vi "LabviewMonitoringApplication - Copy.vi"() -> ()   [LabVIEW 2024]
uses:
  <vilib>/Utility/error.llb/Trim Whitespace One-Sided.vi
  <vilib>/Instr/_visa.llb/VISA Configure Serial Port (Instr).vi
  <vilib>/Utility/file.llb/Read Delimited Spreadsheet (DBL).vi
panel:
  out "all rows":dbl[][](array[numeric])
  out "CONTROL PANEL":enum32{"DASHBOARD", "SERIAL PORT  Settings"}(tab)
  out "Pericol pentru sanatate":u32(colorbox)
  out "Disconfort sever":u32(colorbox)
  out "Disconfort moderat":u32(colorbox)
  out "Usor discomfort":u32(colorbox)
  out "Confortabil":u32(colorbox)
  out "Snapshot data":string
  out "Waveform Chart":T1(graph)
  out "return count read":u32
  in  "STOP":bool=TRUE
  in  "milliseconds to wait":u32=1000
  out "VISA resource name out read":refnum<visa-resource-name>="COM32"
  in  "Start Measurement":bool=TRUE
  out "READ BUFFER":string
  out "Prog. Cnt":i64
  out "AdcValue":dbl
  out "R0 value (kOHm)":dbl(slide) scale=0.0..10.0 scale format="%.2f"
  out "Volatge":dbl(knob) scale=0.0..3.3
  out "Temperature °C":dbl(slide) scale=0.0..100.0 scale format="%#.2g"
  out "Humidity %":dbl(knob) scale=0.1..100.0 scale format="%#.2g"
  out "Heat Index":dbl(slide) scale=0.0..100.0
  out "iPPM_Smoke":i64(slide) scale=0.0..500.0
  out "iPPM_LPG":i64(slide) scale=0.0..100.0
  out "iPPM_CO":i64(slide) scale=0.0..400.0
  in  "Live Data / Historical Data":bool=TRUE
  in  "Temperature":bool=TRUE
  in  "Humidity":bool=TRUE
  in  "PMM_CO":bool=TRUE
  in  "HeatIndex":bool=TRUE
  in  "PMM_LPG":bool=TRUE
  in  "PMM_Smoke":bool=TRUE
  in  "Save file":bool
  in  "Refresh snapshot data":bool
  in  "file path (use dialog)":path
  out "ITU":dbl format="%#.2g"
  in  "file path (dialog if empty)":path
  out "error out read  from VISA":errorcluster={"status"=TRUE, "code"=-1073807339, "source"="VISA Read in LabviewMonitoringApplication.vi"}
  in  "VISA resource name":refnum<visa-resource-name>="COM32"
  in  "Enable Termination\nChar (T)":bool=TRUE
  in  "timeout (ms)":u32=10000
  in  "baud rate (115200)":u32=115200
  in  "byte count":u32=100
  in  "parity (0:none)":enum16{"None", "Odd", "Even", "Mark", "Space"}(ring)
  in  "data bits (8)":u16=8 min=5 max=8 step=1
  in  "termination char\n(0xA = '\\n' = LF)":u8=10 format="%.0x"
  in  "flow control (0:none)":u16(ring) items=["None", "XON/XOFF", "RTS/CTS", "XON/XOFF & RTS/CTS", "DTR/DSR", "XON/XOFF & DTR/DSR"]
  in  "stop bits (10: 1 bit)":u16(ring)=10 items=["1.0"=10, "1.5"=15, "2.0"=20]
  out "error writing file":errorcluster
  out "Snapshot line":string
  # "Select signals (for live data)"
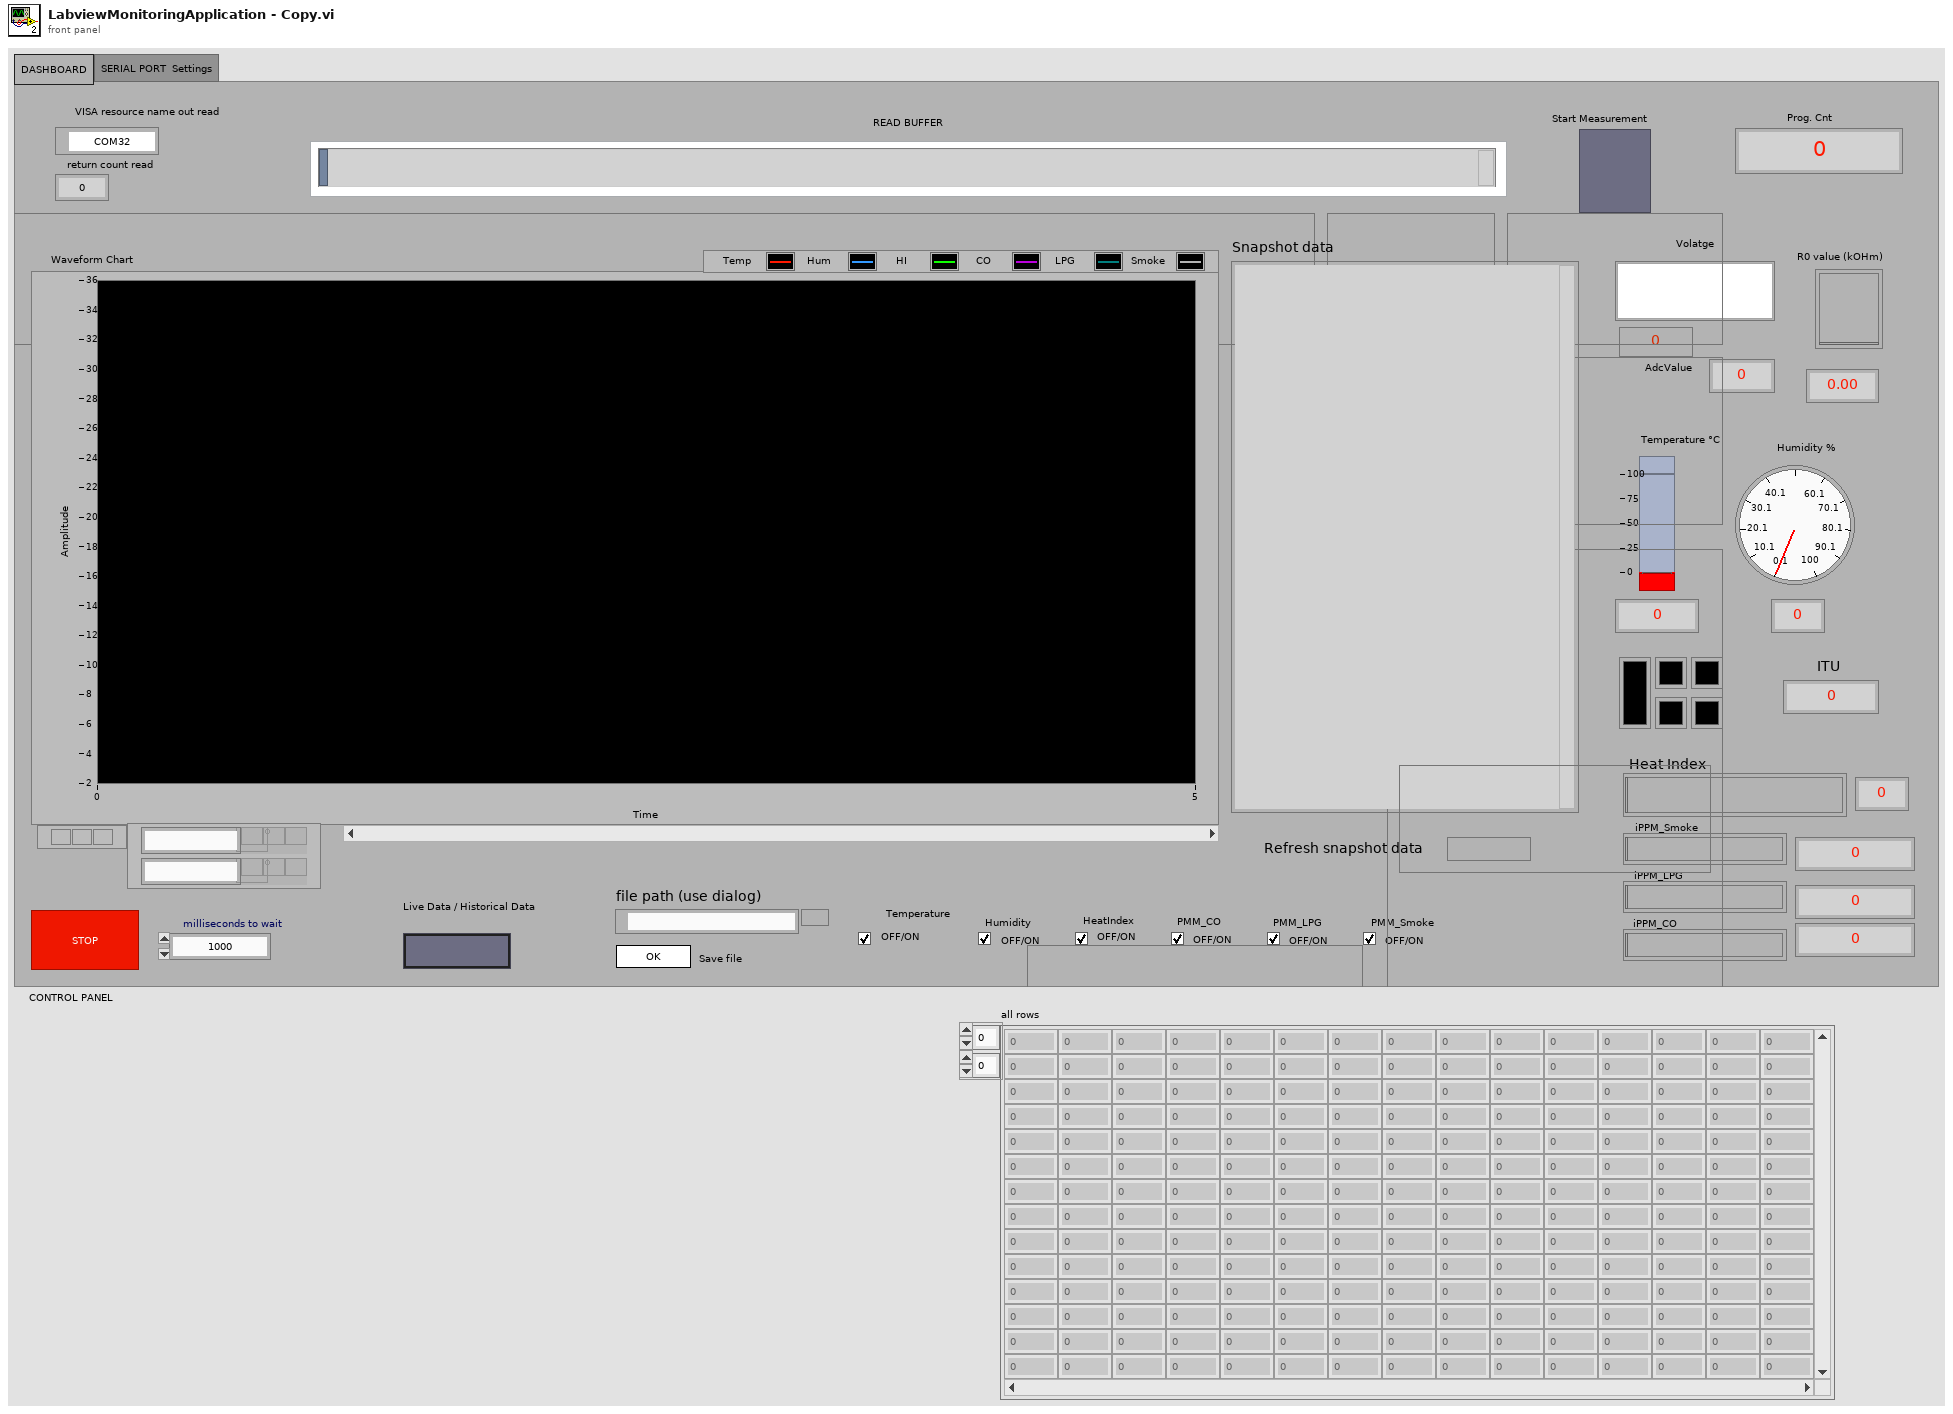
[diagram p1: front panel]
types:
  T1 = cluster{"Temperature °C ":dbl, "Humidity %":dbl, "Heat Index":dbl, "iPPM_CO":dbl, "iPPM_LPG":dbl, "iPPM_Smoke":dbl}
  T2 = enum16{"open", "replace", "create", "open or create", "replace or create", "replace or create with confirmation"}
  T3 = cluster{"Numeric":dbl, "Numeric":dbl, "Numeric":dbl, "Numeric":dbl, "Numeric":dbl, "Numeric":dbl}
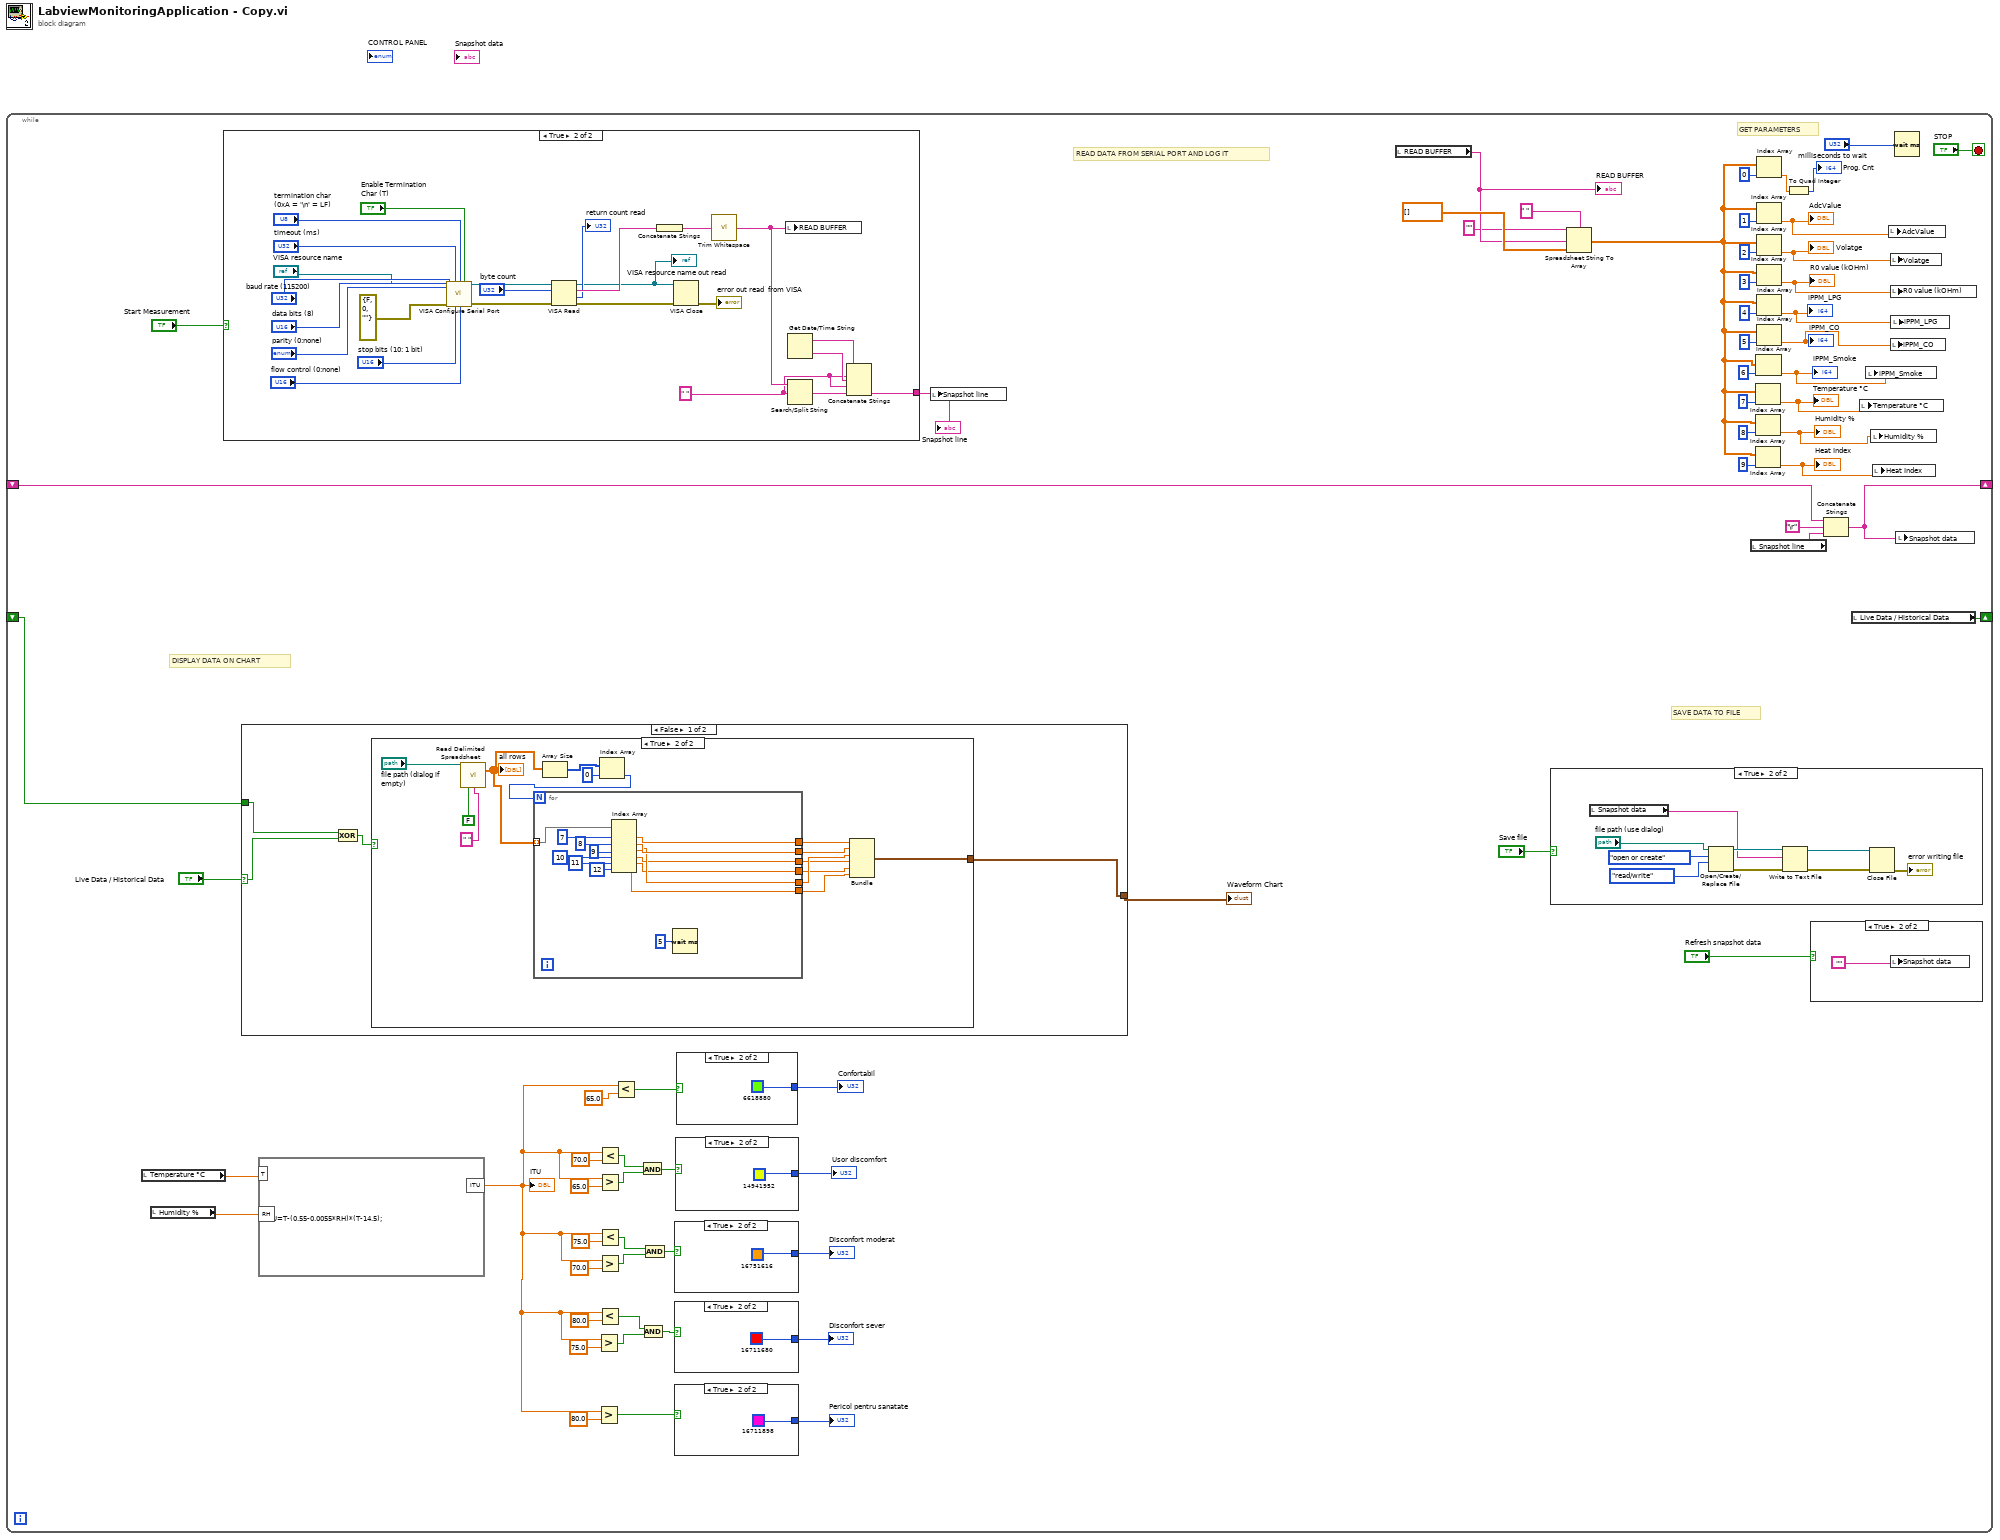
[diagram p0: block diagram]
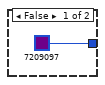
[diagram p2: hidden frame]
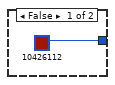
[diagram p3: hidden frame]
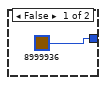
[diagram p4: hidden frame]
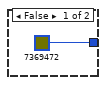
[diagram p5: hidden frame]
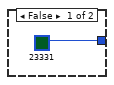
[diagram p6: hidden frame]
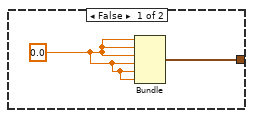
[diagram p9: hidden frame]
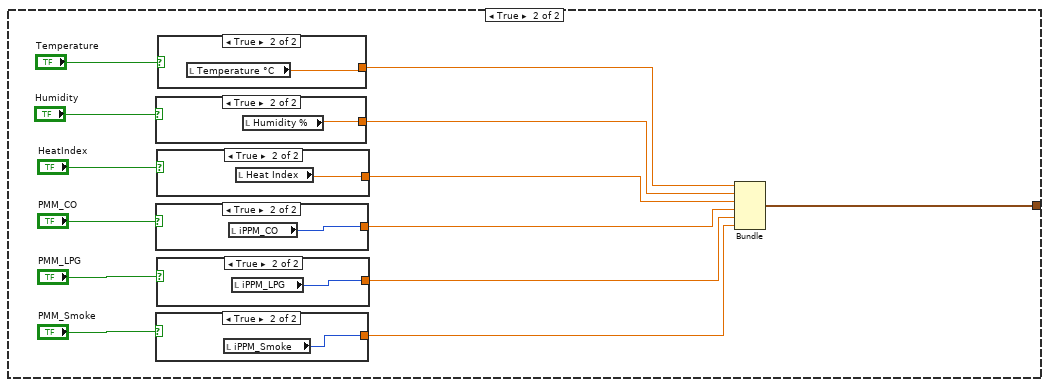
[diagram p10: hidden frame]
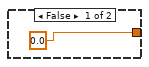
[diagram p11: hidden frame]
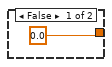
[diagram p12: hidden frame]
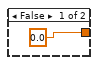
[diagram p13: hidden frame]
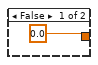
[diagram p14: hidden frame]
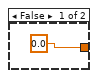
[diagram p15: hidden frame]
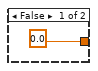
[diagram p16: hidden frame]
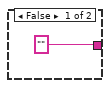
[diagram p17: hidden frame]
diagram:
  n1 = while {
    shift-right: [w33] -> _
    shift-left: _ -> [w34]
    shift-right: [w29] -> _
    shift-left: _ -> [w28]
    stop <- "STOP" stop-if-true
    # "SAVE DATA TO FILE"
    # "DISPLAY DATA ON CHART"
    # "READ DATA FROM SERIAL PORT AND LOG IT"
    # "GET PARAMETERS"
    n2 = local read "Temperature °C"() -> (w26:dbl)
    n3 = local read "Humidity %"() -> (w27:dbl)
    n4 = case shown="True" "Start Measurement" {
      tunnel: ["" w151] -> w31
      frame False {
      }
      frame True {
        w149 = " "
        n5 = call-poly "VISA Configure Serial Port"("VISA resource name"="VISA resource name", "timeout (10sec)"="timeout (ms)", "termination char\n(0xA = '\\n' = LF)"="termination char\n(0xA = '\\n' = LF)", "Enable Termination\nChar (T)"="Enable Termination\nChar (T)", "baud rate (9600)"="baud rate (115200)", "data bits (8)"="data bits (8)", "parity (0:none)"="parity (0:none)", "error in (no error)"=errorcluster {"status"=FALSE, "code"=0, "source"=""}, "stop bits (10: 1 bit)"="stop bits (10: 1 bit)", "flow control (0:none)"="flow control (0:none)") -> ("VISA resource name out"=w165:refnum<visa-resource-name>, "error out"=w164:errorcluster)  [unwired: 4 in]
        n6 = VISA Read(VISA resource name=w165, byte count="byte count", error in (no error)=w164) -> (VISA resource name out=w154:refnum<visa-resource-name>, read buffer=w163:string, return count=→"return count read":u32, error out=w155:errorcluster)
        "VISA resource name out read" <- w154
        n7 = Concatenate Strings(w163) -> (w160:string)
        n8 = VISA Close(VISA resource name=w154, error in (no error)=w155) -> (error out=→"error out read  from VISA":errorcluster)
        n9 = call <vilib>:"Trim Whitespace.vi"("string"=w160) -> ("trimmed string"=w152:string)  [unwired: 1 in]
        n10 = local write "READ BUFFER"(w152) -> ()
        n11 = Search/Split String(string=w152, search string/char (-)=w149) -> (match + rest of string=w153:string)  [unwired: 1 in, 2 out]
        n12 = Get Date/Time String() -> (date string=w148:string, time string=w150:string)  [unwired: 3 in]
        n13 = Concatenate Strings(w148, w149, w150, w149, w153) -> (w151:string)
      }
    }
    "Snapshot line" <- w31
    n14 = case shown="False" "Live Data / Historical Data" {
      selector: "Live Data / Historical Data" -> [w90 _]
      tunnel: [w88 w122] -> w38
      tunnel: w28 -> [w91 _]
      frame False {
        n15 = Exclusive Or(1:w90, 2:w91) -> (0:w89:bool)
        n16 = case shown="True" w89 {
          tunnel: [w93 w94] -> w88
          frame False {
            w92 = 0.0
            n17 = Bundle(w92, w92, w92, w92, w92, w92) -> (w93:cluster{dbl, dbl, dbl, dbl, dbl, dbl})  [unwired: 1 in]
          }
          frame True {
            n18 = call-poly <vilib>:"Read Delimited Spreadsheet.vi"("file path (dialog if empty)"="file path (dialog if empty)", "transpose? (F)"=FALSE, "delimiter (\\t)"=" ") -> ("all rows"=w101:dbl[][])  [unwired: 7 in, 5 out]
            "all rows" <- w101
            n19 = Array Size(array=w101) -> (size(s)=w103:i32[])
            n20 = Index Array(array=w103, index=0) -> (element=w102:i32)
            n21 = for {
              N: w102 -> [_]
              tunnel: w101 -> [w121] mode=indexing
              tunnel: [w114] -> w100
              tunnel: [w113] -> w99
              tunnel: [w112] -> w98
              tunnel: [w111] -> w97
              tunnel: [w110] -> w96
              tunnel: [w109] -> w95
              n22 = Index Array(array=w121, index #1=7 ("index"), index #2=8 ("index"), index #3=9 ("index"), index #4=10 ("index"), index #5=11 ("index"), index #6=12 ("index")) -> (element #1=w114:dbl, element #2=w113:dbl, element #3=w112:dbl, element #4=w111:dbl, element #5=w110:dbl, element #6=w109:dbl)
              n23 = Wait (ms)(milliseconds to wait=u32 5) -> ()  [unwired: 1 out]
            }
            n24 = Bundle("Numeric"=w100, "Numeric"=w99, "Numeric"=w98, "Numeric"=w97, "Numeric"=w96, "Numeric"=w95) -> (w94:T3)  [unwired: 1 in]
          }
        }
      }
      frame True {
        n25 = case shown="True" "Humidity" {
          tunnel: [0.0 w144] -> w127
          frame False {
          }
          frame True {
            n26 = local read "Humidity %"() -> (w144:dbl)
          }
        }
        n27 = case shown="True" "PMM_CO" {
          tunnel: [0.0 w140] -> w125
          frame False {
          }
          frame True {
            n28 = local read "iPPM_CO"() -> (w140:i64)
          }
        }
        n29 = case shown="True" "PMM_Smoke" {
          tunnel: [0.0 w136] -> w123
          frame False {
          }
          frame True {
            n30 = local read "iPPM_Smoke"() -> (w136:i64)
          }
        }
        n31 = case shown="True" "HeatIndex" {
          tunnel: [0.0 w142] -> w126
          frame False {
          }
          frame True {
            n32 = local read "Heat Index"() -> (w142:dbl)
          }
        }
        n33 = case shown="True" "PMM_LPG" {
          tunnel: [0.0 w138] -> w124
          frame False {
          }
          frame True {
            n34 = local read "iPPM_LPG"() -> (w138:i64)
          }
        }
        n35 = case shown="True" "Temperature" {
          tunnel: [0.0 w146] -> w133
          frame False {
          }
          frame True {
            n36 = local read "Temperature °C"() -> (w146:dbl)
          }
        }
        n37 = Bundle("Temperature °C"=w133, "Humidity %"=w127, "Heat Index"=w126, "iPPM_CO"=w125, "iPPM_LPG"=w124, "iPPM_Smoke"=w123) -> (w122:T1)  [unwired: 1 in]
      }
    }
    "Waveform Chart" <- w38
    n38 = formula code="ITU=T-(0.55-0.0055*RH)*(T-14.5);"("T"=w26, "RH"=w27) -> ("ITU"=w1:dbl)
    "ITU" <- w1
    n39 = Greater?(x=w1, y=75.0) -> (0:w13:bool)
    n40 = Greater?(x=w1, y=80.0) -> (0:w18:bool)
    n41 = Greater?(x=w1, y=65.0) -> (0:w10:bool)
    n42 = Greater?(x=w1, y=70.0) -> (0:w12:bool)
    n43 = Less?(x=w1, y=80.0) -> (x < y?=w14:bool)
    n44 = Less?(x=w1, y=70.0) -> (x < y?=w9:bool)
    n45 = Less?(x=w1, y=75.0) -> (x < y?=w11:bool)
    n46 = Less?(x=w1, y=65.0 ("x")) -> (x < y?=w25:bool)
    n47 = And(x=w9, y=w10) -> (x .and. y?=w17:bool)
    n48 = And(x=w14, y=w13) -> (x .and. y?=w15:bool)
    n49 = And(x=w11, y=w12) -> (x .and. y?=w16:bool)
    n50 = case shown="True" w16 {
      tunnel: [u32 8999936 ("Pericol pentru sanatate 2") u32 16751616 ("Pericol pentru sanatate 2")] -> w21
      frame False {
      }
      frame True {
      }
    }
    "Disconfort moderat" <- w21
    n51 = case shown="True" w15 {
      tunnel: [u32 10426112 ("Pericol pentru sanatate 2") u32 16711680 ("Pericol pentru sanatate 2")] -> w22
      frame False {
      }
      frame True {
      }
    }
    "Disconfort sever" <- w22
    n52 = case shown="True" w18 {
      tunnel: [u32 7209097 ("Pericol pentru sanatate 2") u32 16711898 ("Pericol pentru sanatate 2")] -> w23
      frame False {
      }
      frame True {
      }
    }
    "Pericol pentru sanatate" <- w23
    n53 = case shown="True" w17 {
      tunnel: [u32 7369472 ("Pericol pentru sanatate 2") u32 14941952 ("Pericol pentru sanatate 2")] -> w20
      frame False {
      }
      frame True {
      }
    }
    "Usor discomfort" <- w20
    n54 = case shown="True" w25 {
      tunnel: [u32 23331 ("Pericol pentru sanatate 2") u32 6618880 ("Pericol pentru sanatate 2")] -> w24
      frame False {
      }
      frame True {
      }
    }
    "Confortabil" <- w24
    n55 = local write "Snapshot line"(w31) -> ()
    n56 = local read "READ BUFFER"() -> (w63:string)
    "READ BUFFER" <- w63
    n57 = case shown="True" "Save file" {
      frame False {
      }
      frame True {
        n58 = local read "Snapshot data"() -> (w81:string)
        n59 = Open/Create/Replace File(file path (use dialog)="file path (use dialog)", operation (0:open)=T2."open or create", access (0:read/write)=enum16{"read/write", "read-only", "write-only"}."read/write") -> (refnum out=w86:refnum<file>, error out=w85:errorcluster)  [unwired: 3 in, 1 out]
        n60 = Write to Text File(file (use dialog)=w86, text=w81, error in=w85) -> (refnum out=w83:refnum<file>, error out=w84:errorcluster)  [unwired: 1 in, 1 out]
        n61 = Close File(refnum=w83, error in=w84) -> (error out=→"error writing file":errorcluster)  [unwired: 1 out]
      }
    }
    n62 = Spreadsheet String To Array(delimiter (Tab)=" ", format string="", spreadsheet string=w63, array type (2D Dbl)=dbl[] []) -> (array=w49:dbl[])
    n63 = local read "Snapshot line"() -> (w30:string)
    n64 = Index Array(array=w49, index=7) -> (element=w41:dbl)
    "Temperature °C" <- w41
    n65 = Index Array(array=w49, index=8) -> (element=w42:dbl)
    "Humidity %" <- w42
    n66 = Index Array(array=w49, index=9) -> (element=w43:dbl)
    "Heat Index" <- w43
    n67 = Index Array(array=w49, index=6) -> (element=w40:dbl)
    "iPPM_Smoke" <- w40
    n68 = Index Array(array=w49, index=0) -> (element=w60:dbl)
    n69 = Index Array(array=w49, index=1) -> (element=w48:dbl)
    "AdcValue" <- w48
    n70 = Index Array(array=w49, index=2) -> (element=w47:dbl)
    "Volatge" <- w47
    n71 = Index Array(array=w49, index=3) -> (element=w46:dbl)
    "R0 value (kOHm)" <- w46
    n72 = Index Array(array=w49, index=4) -> (element=w45:dbl)
    "iPPM_LPG" <- w45
    n73 = Index Array(array=w49, index=5) -> (element=w44:dbl)
    "iPPM_CO" <- w44
    n74 = To Quad Integer(1:w60) -> (0:→"Prog. Cnt":i64)
    n75 = case shown="True" "Refresh snapshot data" {
      frame False {
      }
      frame True {
        n76 = local write "Snapshot data"("") -> ()
      }
    }
    n77 = Concatenate Strings(w34, "\r", w30) -> (w33:string)
    n78 = local read "Live Data / Historical Data"() -> (w29:bool)
    n79 = local write "Temperature °C"(w41) -> ()
    n80 = local write "iPPM_Smoke"(w40) -> ()
    n81 = local write "Humidity %"(w42) -> ()
    n82 = local write "Heat Index"(w43) -> ()
    n83 = local write "AdcValue"(w48) -> ()
    n84 = local write "Volatge"(w47) -> ()
    n85 = local write "R0 value (kOHm)"(w46) -> ()
    n86 = local write "iPPM_CO"(w44) -> ()
    n87 = local write "iPPM_LPG"(w45) -> ()
    n88 = Wait (ms)(milliseconds to wait="milliseconds to wait") -> ()  [unwired: 1 out]
    n89 = local write "Snapshot data"(w33) -> ()
  }
